vi "Parse Config to Queue.vi"(8 "error in":errorcluster, 11 "DSF Configuration Session in":T1) -> (0 "error out":errorcluster, 3 "DSF Configuration Session out":T1)   [LabVIEW 2017, in "DSF Configuration API.lvlib"]
uses:
  DSF Configuration API.lvlib
  Controls/Session/DSF Configuration Reference.ctl
  Controls/DSF File Format/Internal.DSF Configuration.ctl
  Public/Controls/DSF Version Info.ctl
  Controls/DSF File Format/Internal.DSF Plugin with ID.ctl
  Controls/DSF File Format/Internal.DSF Plugin Info.ctl
  Public/Controls/DSF Timing Info.ctl
  Controls/DSF File Format/Internal.DSF Group with ID.ctl
  Controls/DSF File Format/Internal.DSF Group Info.ctl
  Controls/DSF File Format/Internal.DSF Transfer with ID.ctl
  Controls/DSF File Format/Internal.DSF Transfer Info.ctl
  Controls/DSF File Format/Internal.DSF Channel with ID.ctl
  Controls/DSF File Format/Internal.DSF Channel Info.ctl
  Controls/DSF File Format/Internal.DSF Settings with ID.ctl
  Controls/DSF File Format/Internal.DSF Settings Info.ctl
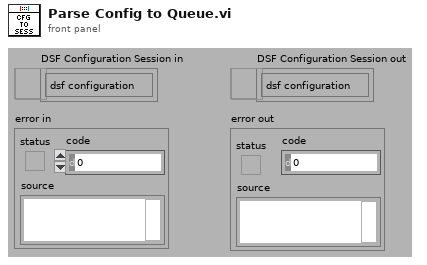
[diagram p1: front panel]
types:
  T1 = typedef "DSF Configuration API.lvlib/DSF Configuration Reference.ctl" = refnum<data-value>
  T2 = typedef "DSF Configuration API.lvlib/Internal.DSF Configuration.ctl" = cluster{"dsfversion":T3, "version":T3, "plugins":T4[], "groups":T7[], "transfers":T9[], "channels":T11[], "settings":T13[]}
  T3 = typedef "DSF Configuration API.lvlib/DSF Version Info.ctl" = cluster{"major":u32, "minor":u32, "fix":u32, "build":string}
  T4 = typedef "DSF Configuration API.lvlib/Internal.DSF Plugin with ID.ctl" = cluster{"id":string, "values":T5}
  T5 = typedef "DSF Configuration API.lvlib/Internal.DSF Plugin Info.ctl" = cluster{"type":string, "timing":T6, "group ids":string[], "settings id":string}
  T6 = typedef "DSF Configuration API.lvlib/DSF Timing Info.ctl" = cluster{"priority":i32, "decimation":i32, "offset":i32}
  T7 = typedef "DSF Configuration API.lvlib/Internal.DSF Group with ID.ctl" = cluster{"id":string, "values":T8}
  T8 = typedef "DSF Configuration API.lvlib/Internal.DSF Group Info.ctl" = cluster{"direction":i32, "timing":T6, "transfer ids":string[], "settings id":string}
  T9 = typedef "DSF Configuration API.lvlib/Internal.DSF Transfer with ID.ctl" = cluster{"id":string, "values":T10}
  T10 = typedef "DSF Configuration API.lvlib/Internal.DSF Transfer Info.ctl" = cluster{"byte order":i32, "channel ids":string[], "settings id":string}
  T11 = typedef "DSF Configuration API.lvlib/Internal.DSF Channel with ID.ctl" = cluster{"id":string, "values":T12}
  T12 = typedef "DSF Configuration API.lvlib/Internal.DSF Channel Info.ctl" = cluster{"count":i32, "offset":i32, "data type":i32, "resource path":string, "settings id":string}
  T13 = typedef "DSF Configuration API.lvlib/Internal.DSF Settings with ID.ctl" = cluster{"id":string, "values":T14}
  T14 = typedef "DSF Configuration API.lvlib/Internal.DSF Settings Info.ctl" = cluster{"key":string, "value":string}[]
  T15 = cluster{"dsf configuration":T2, "path":path, "dirty":bool}
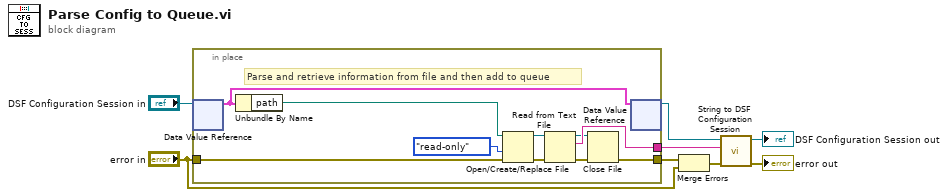
[diagram p0: block diagram]
diagram:
  n1 = in-place {
    in-place-border: [w17] -> w7
    in-place-border: "error in" -> [w11]
    in-place-border: [w10] -> w4
    # "Parse and retrieve information from file and then add to queue"
    n2 = in-place-dvr #1("DSF Configuration Session in") -> (w9:T15)  [unwired: 1 out]
    n3 = Unbundle By Name(w9) -> ("path"=w18:path)
    n4 = Open/Create/Replace File(file path (use dialog)=w18, error in=w11, access (0:read/write)=enum16{"read/write", "read-only", "write-only"}."read-only") -> (refnum out=w16:refnum<file>, error out=w15:errorcluster)  [unwired: 4 out]
    n5 = Read from Text File(file (use dialog)=w16, error in=w15) -> (refnum out=w13:refnum<file>, text=w17:string, error out=w12:errorcluster)  [unwired: 3 out]
    n6 = Close File(refnum=w13, error in=w12) -> (error out=w10:errorcluster)  [unwired: 1 out]
    n7 = in-place-dvr #1(w9) -> (w1:T1)  [unwired: 1 out]
  }
  n8 = Merge Errors(w4, "error in") -> (w3:errorcluster)
  n9 = call "String to DSF Configuration Session.vi"("error in (no error)"=w3, "string input"=w7, "DSF Configuration Session in"=w1) -> ("error out"=→"error out":errorcluster, "DSF Configuration Session out"=→"DSF Configuration Session out":T1)  [unwired: 7 out]
